vi "_unittest Report.vi"(8 "error in (no error)":errorcluster, 9 "Show Passed? (F)":bool) -> (0 "error out":errorcluster, 2 "All Passed?":bool, 3 "Full Report":string)   [LabVIEW 2019, in "labview_json_tests.lvlib"]
uses:
  labview_json_tests.lvlib
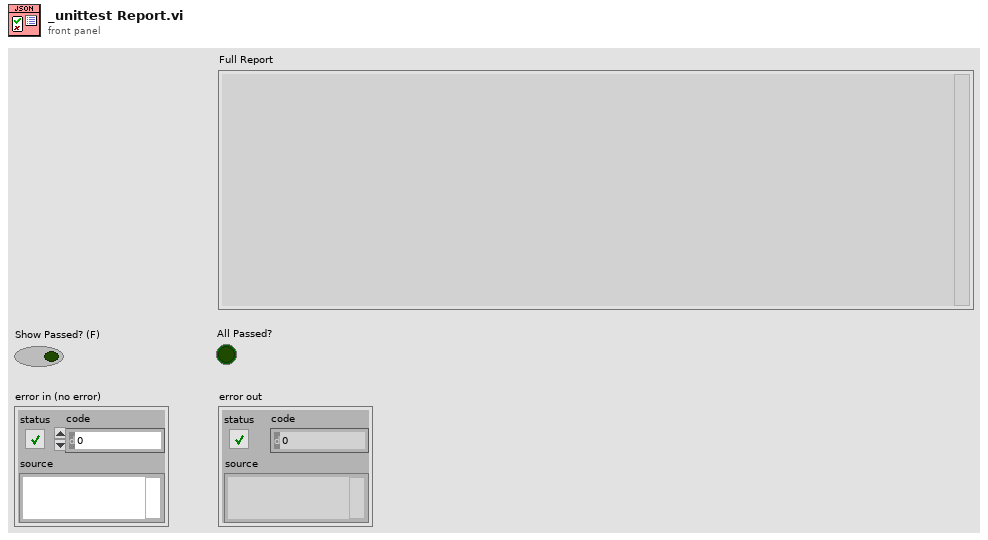
[diagram p1: front panel]
types:
  T1 = enum8{"Report", "Add Test Group", "Add Test Case"}
  T2 = cluster{"Indent":i32[], "VI":string, "TestGroup":string, "Tests":cluster{"Test":string, "Passed":bool, "Info":string}[]}[]
  T3 = cluster{"Test":string, "Passed":bool, "Info":string}[]
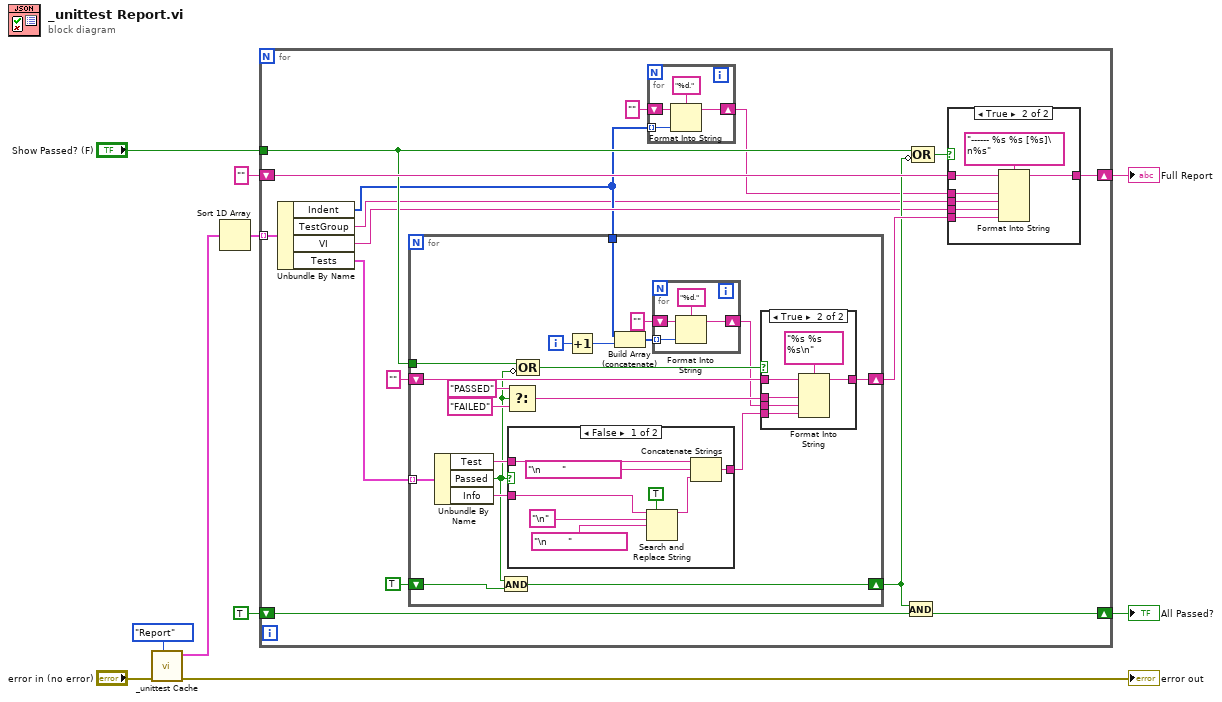
[diagram p0: block diagram]
diagram:
  n1 = call "_unittest Cache.vi"("Action"=T1."Report", "error in (no error)"="error in (no error)") -> ("error out"=→"error out":errorcluster, "Tests"=w2:T2)  [unwired: 8 in]
  n2 = Sort 1D Array(array=w2) -> (sorted array=w1:T2)
  n3 = for {
    tunnel: w1 -> [w27] mode=indexing
    shift-right: [w24] -> w4
    shift-left: "" -> [w25]
    shift-right: [w22] -> w5
    shift-left: TRUE -> [w21]
    tunnel: "Show Passed? (F)" -> [w18]
    n4 = Unbundle By Name(w27) -> ("Indent"=w13:i32[], "TestGroup"=w12:string, "VI"=w14:string, "Tests"=w11:T3)
    n5 = for {
      tunnel: w11 -> [w59] mode=indexing
      shift-right: [w55] -> w20
      shift-left: "" -> [w52]
      shift-right: [w54] -> w19
      shift-left: TRUE -> [w53]
      tunnel: w18 -> [w47]
      tunnel: w13 -> [w45]
      i -> [w41]
      n6 = Unbundle By Name(w59) -> ("Test"=w58:string, "Passed"=w48:bool, "Info"=w57:string)
      n7 = And(x=w48, y=w53) -> (x .and. y?=w54:bool)
      n8 = Select(t="PASSED", s=w48, f="FAILED") -> (s? t:f=w49:string)
      n9 = case shown="False" w48 {
        tunnel: w58 -> [w78 w79]
        tunnel: w57 -> [w74 _]
        tunnel: [w76 w79] -> w56
        frame False {
          n10 = Search and Replace String(replace all?=TRUE ("replace all? (F)"), input string=w74, search string="\n" ("string"), replace string="\n       " ("string")) -> (result string=w75:string)  [unwired: 4 in, 3 out]
          n11 = Concatenate Strings(w78, "\n       " ("string"), w75) -> (w76:string)
        }
        frame True {
        }
      }
      n12 = Compound Arithmetic op=OR(w47, invert w48) -> (w46:bool)
      n13 = Increment(x=w41) -> (x+1=w40:i32)
      n14 = Build Array (concatenate)(w45, w40) -> (w42:i32[])
      n15 = for {
        tunnel: w42 -> [w63] mode=indexing
        shift-right: [w61] -> w43
        shift-left: "" -> [w60]
        n16 = Format Into String(format string="%d.", initial string=w60, w63) -> (resulting string=w61:string)  [unwired: 1 in, 1 out]
      }
      n17 = case shown="True" w46 {
        tunnel: w56 -> [_ w70]
        tunnel: [w64 w69] -> w55
        tunnel: w52 -> [w64 w68]
        tunnel: w43 -> [_ w66]
        tunnel: w49 -> [_ w65]
        frame False {
        }
        frame True {
          n18 = Format Into String(format string="%s %s %s\n", initial string=w68, w65, w66, w70) -> (resulting string=w69:string)  [unwired: 1 in, 1 out]
        }
      }
    }
    n19 = for {
      tunnel: w13 -> [w31] mode=indexing
      shift-right: [w29] -> w15
      shift-left: "" -> [w28]
      n20 = Format Into String(format string="%d.", initial string=w28, w31) -> (resulting string=w29:string)  [unwired: 1 in, 1 out]
    }
    n21 = And(x=w19, y=w21) -> (x .and. y?=w22:bool)
    n22 = Compound Arithmetic op=OR(w18, invert w19) -> (w17:bool)
    n23 = case shown="True" w17 {
      tunnel: w25 -> [w32 w39]
      tunnel: w12 -> [_ w38]
      tunnel: [w32 w36] -> w24
      tunnel: w14 -> [_ w35]
      tunnel: w20 -> [_ w34]
      tunnel: w15 -> [_ w33]
      frame False {
      }
      frame True {
        n24 = Format Into String(format string="------ %s %s [%s]\n%s", initial string=w39, w33, w38, w35, w34) -> (resulting string=w36:string)  [unwired: 1 in, 1 out]
      }
    }
  }
  "Full Report" <- w4
  "All Passed?" <- w5
